vi "test Signed and Unsigned.vi"(8 "error in (no error)":errorcluster, 11 "TestCase in":refnum<class "BCD.lvclass">) -> (0 "error out":errorcluster, 3 "TestCase out":refnum<class "BCD.lvclass">)   [LabVIEW 2027, in "BCD.lvclass"]
uses:
  BCD.lvclass
  f2733c54-cb77-423d-8059-cbd7df94c12a.vi
  079ecff3-6de1-4111-8ef3-12bd571ec372.vi
  2f100830-ea7a-40a1-aee0-f461a025289f.vi
  e6c83ec4-7129-44fe-87e4-b449e3b4cd07.vi
  f2733c54-cb77-423d-8059-cbd7df94c12a.vi/136dcdcb-2dd3-4a4d-a796-a8f7a3f8e1ac.vi
  f2733c54-cb77-423d-8059-cbd7df94c12a.vi/a54b505c-1216-4ef4-8378-3ceda9d188df.vi
  079ecff3-6de1-4111-8ef3-12bd571ec372.vi/136dcdcb-2dd3-4a4d-a796-a8f7a3f8e1ac.vi
  079ecff3-6de1-4111-8ef3-12bd571ec372.vi/a54b505c-1216-4ef4-8378-3ceda9d188df.vi
  2f100830-ea7a-40a1-aee0-f461a025289f.vi/136dcdcb-2dd3-4a4d-a796-a8f7a3f8e1ac.vi
  2f100830-ea7a-40a1-aee0-f461a025289f.vi/a54b505c-1216-4ef4-8378-3ceda9d188df.vi
  e6c83ec4-7129-44fe-87e4-b449e3b4cd07.vi/0a001d06-2809-4638-8d0b-e017d2157007.vi
  e6c83ec4-7129-44fe-87e4-b449e3b4cd07.vi/e08d08e5-79bf-42ec-a5e5-c4db927cd1a5.vi
  Source/Get Bits Per Digit from Base.vi
  C:/Program Files/National Instruments/LabVIEW 2027/vi.lib/addons/_JKI Toolkits/VI Tester/TestCase.llb/TestCase.lvclass
  <vilib>/addons/_JKI Toolkits/VI Tester/TestCase.llb/TestCase.lvclass
panel:
  out "BCD encoded value":bool[](array[boolean])
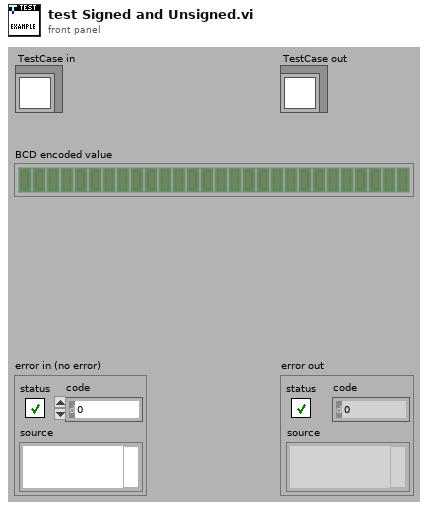
[diagram p1: front panel]
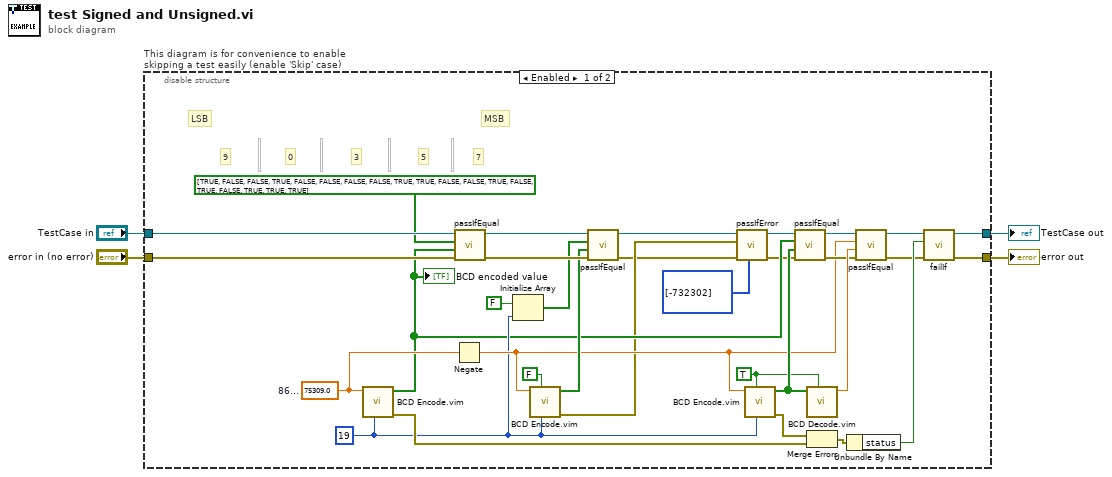
[diagram p0: block diagram]
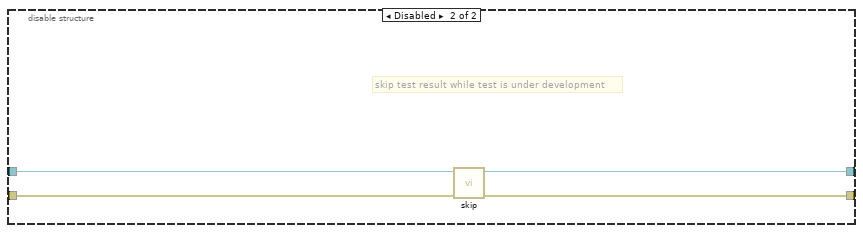
[diagram p2: hidden frame]
diagram:
  n1 = disable-structure "This diagram is for convenience to enable skipping a test easily (enable 'Skip' case)" shown="Enabled" {
    disable-tunnel: "TestCase in" -> [w33 w40]
    disable-tunnel: [w18 w38] -> w1
    disable-tunnel: [w19 w39] -> w3
    disable-tunnel: "error in (no error)" -> [w31 w37]
    frame Enabled {
      w16 = TRUE ("signed")
      w13 = 19 ("data size (bits)")
      w14 = 75309.0  # 86...
      # "MSB"
      # "LSB"
      # "9"
      # "0"
      # "3"
      # "5"
      # "7"
      n2 = call "BCD Encode.vim"("data size (bits)"=w13, "value"=w14) -> ("error out"=w24:errorcluster, "BCD encoded value"=w11:bool[])  [unwired: 7 in, 1 out]
      "BCD encoded value" <- w11
      n3 = Negate(x=w14) -> (-x=w17:dbl)
      n4 = call-dynamic "passIfEqual.vi"("error in (no error)"=w31, "y"=w11, "x"=bool[] [TRUE, FALSE, FALSE, TRUE, FALSE, FALSE, FALSE, FALSE, TRUE, TRUE, FALSE, FALSE, TRUE, FALSE, TRUE, FALSE, TRUE, TRUE, TRUE] ("BCD encoded value"), "TestCase in"=w33) -> ("error out"=w32:errorcluster, "TestCase out"=w34:refnum<class "BCD.lvclass">)  [unwired: 6 in]
      n5 = Initialize Array(FALSE, w13) -> (w12:bool[])
      n6 = call "BCD Encode.vim"("data size (bits)"=w13, "signed"=FALSE, "value"=w17) -> ("error out"=w10:errorcluster, "BCD encoded value"=w29:bool[])  [unwired: 6 in, 1 out]
      n7 = call-dynamic "passIfEqual.vi"("error in (no error)"=w32, "y"=w29, "x"=w12, "TestCase in"=w34) -> ("error out"=w8:errorcluster, "TestCase out"=w9:refnum<class "BCD.lvclass">)  [unwired: 6 in]
      n8 = call-dynamic "passIfError.vi"("passing error codes (default = any error code)"=i32[] [-732302], "error in (no error)"=w8, "error"=w10, "TestCase in"=w9) -> ("error out"=w6:errorcluster, "TestCase out"=w7:refnum<class "BCD.lvclass">)  [unwired: 6 in]
      n9 = call "BCD Encode.vim"("data size (bits)"=w13, "signed"=w16, "value"=w17) -> ("error out"=w25:errorcluster, "BCD encoded value"=w30:bool[])  [unwired: 6 in, 1 out]
      n10 = call-dynamic "passIfEqual.vi"("error in (no error)"=w6, "y"=w30, "x"=w11, "TestCase in"=w7) -> ("error out"=w27:errorcluster, "TestCase out"=w28:refnum<class "BCD.lvclass">)  [unwired: 6 in]
      n11 = call "BCD Decode.vim"("signed"=w16, "BCD encoded value"=w30) -> ("value"=w35:dbl)  [unwired: 9 in]
      n12 = Merge Errors(w25, w24) -> (w23:errorcluster)
      n13 = Unbundle By Name(w23) -> ("status"=w22:bool)
      n14 = call-dynamic "passIfEqual.vi"("error in (no error)"=w27, "y"=w35, "x"=w17, "TestCase in"=w28) -> ("error out"=w20:errorcluster, "TestCase out"=w21:refnum<class "BCD.lvclass">)  [unwired: 6 in]
      n15 = call-dynamic "failIf.vi"("error in (no error)"=w20, "fail"=w22, "TestCase in"=w21) -> ("error out"=w19:errorcluster, "TestCase out"=w18:refnum<class "BCD.lvclass">)  [unwired: 7 in]
    }
    frame Disabled {
      # "skip test result while test is under development"
      n16 = call <vilib>:"skip.vi"("error in (no error)"=w37, "TestCase in"=w40) -> ("error out"=w39:errorcluster, "TestCase out"=w38:refnum<class "BCD.lvclass">)  [unwired: 8 in]
    }
  }
  "error out" <- w3
  "TestCase out" <- w1
